vi "isComplete.vi"(8 "error in (no error)":errorcluster, 11 "Mission in":refnum<class "GenericMission.lvclass">) -> (0 "error out":errorcluster, 2 "Mission Complete?":bool, 3 "Mission out":refnum<class "GenericMission.lvclass">)   [LabVIEW 2011, in "GenericMission.lvclass"]
doc: "Determine whether or not a mission is complete.\n\nNote: This is a dynamic dispatch method of GenericMission. The correct method will be called based on the run-time class of this object, a child class of GenericMission.\n\nAuthor: Jared Kirschner"
uses:
  GenericMission.lvclass
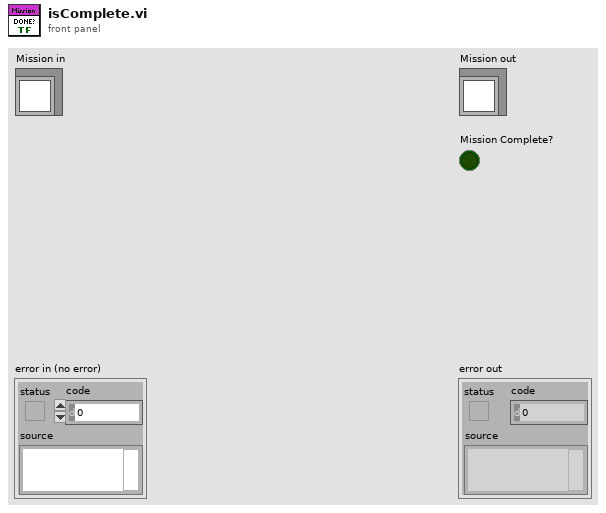
[diagram p1: front panel]
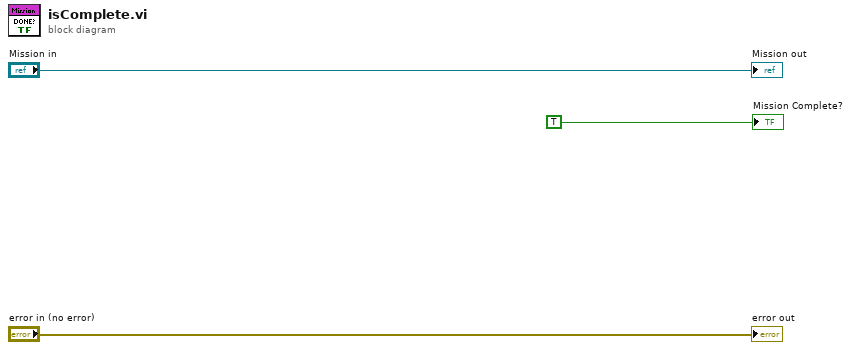
[diagram p0: block diagram]
diagram:
  "error out" <- "error in (no error)"
  "Mission out" <- "Mission in"
  "Mission Complete?" <- TRUE ("Mission Complete?")
